vi "SRX_Reset Select.vi"(8 "Error":errorcluster, 9 "Reset Select":T1, 11 "PhoenixMotorControlDevRef":T2={"DeviceStatus"={"status"=FALSE, "code"=0, "source"=""}, "Type"=enum."PWM", "PWM"={"PWM Channel"=enum."PWM 1", "DeadBand"={"Name"="", "maxPositivePwm"=0, "minPositivePwm"=0, "centerPwm"=0, "maxNegativePwm"=0, "minNegativePwm"=0, "angularRange"=0}}, "CAN"={"Device Number"=0, "SetOutput VI Ref"=variant(enum8{"Percent VBus", "Current", "Speed", "Position", "Voltage"} enum."Percent VBus"), "GetOutput VI Ref"=variant(refnum<k1> refnum), "Enable VI Ref"=variant(dbl 12.0), "Disable VI Ref"=variant(enum8{"Percent VBus", "Speed", "Position", "Slave", "Unchanged / Invalid", "Voltage Compensation", "Current", "Motion Profile"} enum."Percent VBus"), "Data"=variant}, "Invert"=FALSE, "DIO PWM"={"PWM \"Enable\" Channel"=enum."Invalid", "DIOChannel"=enum."Invalid", "PWM Rate"=0.0}}) -> (0 "Error Out":errorcluster, 3 "PhoenixMotorControlDevRef Out":T2={"DeviceStatus"={"status"=FALSE, "code"=0, "source"=""}, "Type"=enum."PWM", "PWM"={"PWM Channel"=enum."Invalid", "DeadBand"={"Name"="", "maxPositivePwm"=0, "minPositivePwm"=0, "centerPwm"=0, "maxNegativePwm"=0, "minNegativePwm"=0, "angularRange"=0}}, "CAN"={"Device Number"=0, "SetOutput VI Ref"=variant(enum8{"Percent VBus", "Current", "Speed", "Position", "Voltage"} enum."Percent VBus"), "GetOutput VI Ref"=variant(refnum<k1> refnum), "Enable VI Ref"=variant(dbl 12.0), "Disable VI Ref"=variant(enum8{"Percent VBus", "Speed", "Position", "Slave", "Unchanged / Invalid", "Voltage Compensation", "Current", "Motion Profile"} enum."Percent VBus"), "Data"=variant}, "Invert"=FALSE, "DIO PWM"={"PWM \"Enable\" Channel"=enum."Invalid", "DIOChannel"=enum."Invalid", "PWM Rate"=0.0}})   [LabVIEW 2017]
uses:
  <vilib>/Rock Robotics/WPI/MotorControl/WPI_MotorControlDeviceRef.ctl
  <vilib>/Rock Robotics/WPI/MotorControl/WPI_MotorControlType.ctl
  <vilib>/Rock Robotics/SystemInterfaces/DIO/FPGA_DIOPWMChannel.ctl
  <vilib>/Rock Robotics/WPI/PWM/WPI_PWMDeadband.ctl
  <vilib>/Rock Robotics/SystemInterfaces/DIO/FPGA_DIOChannel.ctl
  TypeDefs SRX/ENUM_SRX_Reset Select.ctl
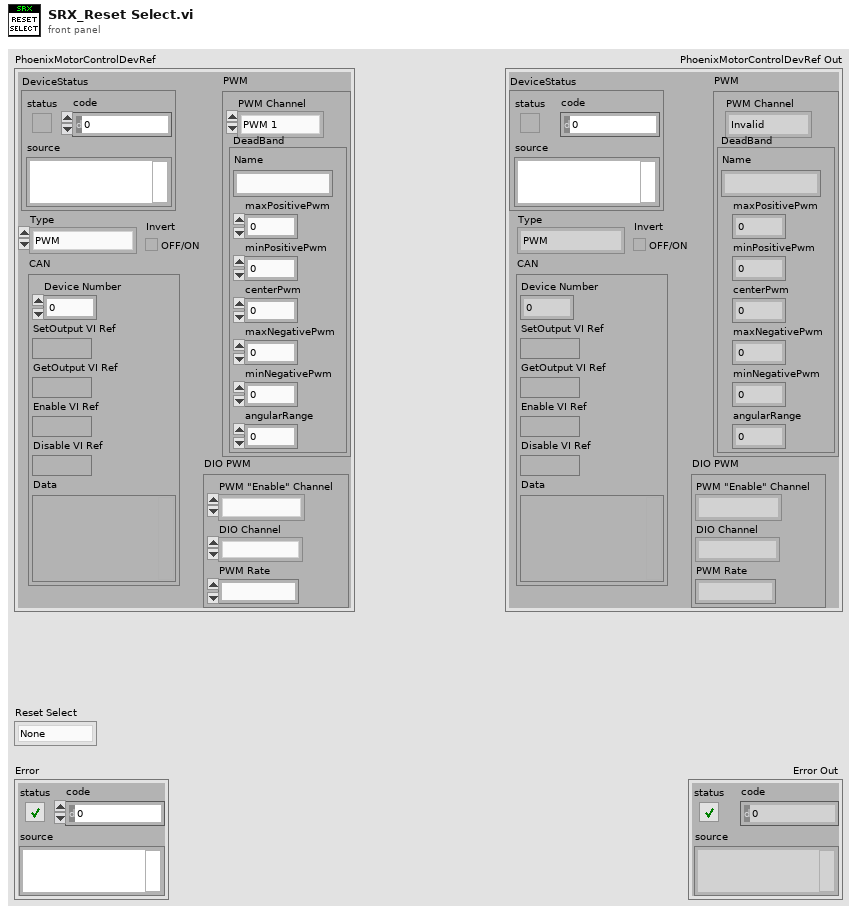
[diagram p1: front panel]
types:
  T1 = typedef "ENUM_SRX_Reset Select.ctl" = enum16{"None", "Sensor", "I-Accum", "Sticky Faults", "ALL"}
  T2 = typedef "WPI_MotorControlDeviceRef.ctl" = cluster{"DeviceStatus":errorcluster, "Type":T3, "PWM":cluster{"PWM Channel":T4, "DeadBand":T5}, "CAN":cluster{"Device Number":u8, "SetOutput VI Ref":variant, "GetOutput VI Ref":variant, "Enable VI Ref":variant, "Disable VI Ref":variant, "Data":variant}, "Invert":bool, "DIO PWM":cluster{"PWM \"Enable\" Channel":T4, "DIOChannel":T6, "PWM Rate":dbl}}
  T3 = typedef "WPI_MotorControlType.ctl" = enum16{"PWM", "CAN", "DIO PWM"}
  T4 = typedef "FPGA_DIOPWMChannel.ctl" = enum8{"PWM 0", "PWM 1", "PWM 2", "PWM 3", "PWM 4", "PWM 5", "PWM 6", "PWM 7", "PWM 8", "PWM 9", "PWM MXP 0", "PWM MXP 1", "PWM MXP 2", "PWM MXP 3", "PWM MXP 4", "PWM MXP 5", "PWM MXP 6", "PWM MXP 7", "PWM MXP 8", "PWM MXP 9", "Invalid"}
  T5 = typedef "WPI_PWMDeadband.ctl" = cluster{"Name":string, "maxPositivePwm":i32, "minPositivePwm":i32, "centerPwm":i32, "maxNegativePwm":i32, "minNegativePwm":i32, "angularRange":u16}
  T6 = typedef "FPGA_DIOChannel.ctl" = enum8{"DIO 0", "DIO 1", "DIO 2", "DIO 3", "DIO 4", "DIO 5", "DIO 6", "DIO 7", "DIO 8", "DIO 9", "DIO MXP 0", "DIO MXP 1", "DIO MXP 2", "DIO MXP 3", "DIO MXP 4", "DIO MXP 5", "DIO MXP 6", "DIO MXP 7", "DIO MXP 8", "DIO MXP 9", "DIO MXP 10", "DIO MXP 11", "DIO MXP 12", "DIO MXP 13", "DIO MXP 14", "DIO MXP 15", "SPI Port CS1", "SPI Port CS2", "SPI Port CS3", "SPI Port MISO", "SPI Port MOSI", "Invalid"}
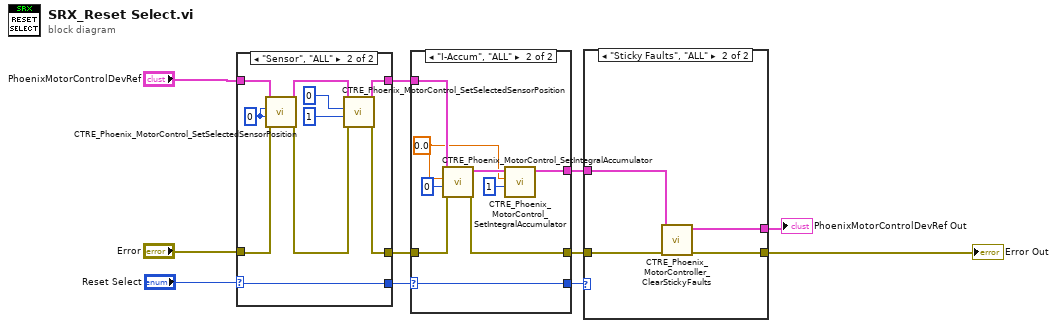
[diagram p0: block diagram]
diagram:
  n1 = case shown="\"Sensor\", \"ALL\"" "Reset Select" {
    selector: "Reset Select" -> [w12 w15]
    tunnel: [w14 w24] -> w11
    tunnel: [w13 w23] -> w6
    tunnel: "PhoenixMotorControlDevRef" -> [w14 w22]
    tunnel: "Error" -> [w13 w20]
    tunnel: [w12 w15] -> w2
    frame Default {
    }
    frame "Sensor", "ALL" {
      w18 = u32 0 ("pidLoopIdx")
      n2 = call "CTRE_Phoenix_MotorControl_SetSelectedSensorPosition.vi"("error in (no error)"=w20, "pidLoopIdx"=w18, "New Sensor Position"=w18, "PhoenixMotorControlDevRef"=w22) -> ("error out"=w19:errorcluster, "PhoenixMotorControlDevRef"=w21:T2)  [unwired: 6 in]
      n3 = call "CTRE_Phoenix_MotorControl_SetSelectedSensorPosition.vi"("error in (no error)"=w19, "pidLoopIdx"=u32 1, "New Sensor Position"=u32 0 ("pidLoopIdx"), "PhoenixMotorControlDevRef"=w21) -> ("error out"=w23:errorcluster, "PhoenixMotorControlDevRef"=w24:T2)  [unwired: 6 in]
    }
  }
  n4 = case shown="\"I-Accum\", \"ALL\"" w2 {
    selector: w2 -> [w26 w33]
    tunnel: w11 -> [w25 w36]
    tunnel: [w25 w30] -> w10
    tunnel: [w27 w35] -> w7
    tunnel: w6 -> [w27 w34]
    tunnel: [w26 w33] -> w1
    frame Default {
    }
    frame "I-Accum", "ALL" {
      w28 = 0.0 ("Integral Accumulator Value")
      n5 = call "CTRE_Phoenix_MotorControl_SetIntegralAccumulator.vi"("Error"=w34, "PidLoopIdx"=u32 0, "Integral Accumulator Value"=w28, "PhoenixMotorControlDevRef"=w36) -> ("Error Out"=w35:errorcluster, "PhoenixMotorControlDevRef Out"=w31:T2)  [unwired: 6 in]
      n6 = call "CTRE_Phoenix_MotorControl_SetIntegralAccumulator.vi"("PidLoopIdx"=u32 1, "Integral Accumulator Value"=w28, "PhoenixMotorControlDevRef"=w31) -> ("PhoenixMotorControlDevRef Out"=w30:T2)  [unwired: 7 in, 1 out]
    }
  }
  n7 = case shown="\"Sticky Faults\", \"ALL\"" w1 {
    tunnel: w10 -> [w38 w42]
    tunnel: [w38 w41] -> w9
    tunnel: [w37 w40] -> w8
    tunnel: w7 -> [w37 w39]
    frame Default {
    }
    frame "Sticky Faults", "ALL" {
      n8 = call "CTRE_Phoenix_MotorController_ClearStickyFaults.vi"("Error"=w39, "PhoenixMotorControlDevRef"=w42) -> ("Error Out"=w40:errorcluster, "PhoenixMotorControlDevRef Out"=w41:T2)  [unwired: 8 in]
    }
  }
  "PhoenixMotorControlDevRef Out" <- w9
  "Error Out" <- w8
